vi "Unregister API.vi"(8 "error in (no error)":errorcluster, 10 "API":refnum<class "API.lvclass">, 11 "VolatusCore in":refnum<class "VolatusCoreTask.lvclass">) -> (0 "error out":errorcluster, 3 "VolatusCore out":refnum<class "VolatusCoreTask.lvclass">)   [LabVIEW 2020, in "Volatus.lvlib" / "VolatusCoreTask.lvclass"]
uses:
  VolatusCoreTask.lvclass
  API/API.lvclass
  VolatusCoreTask.lvclass/VolatusCoreTask.ctl
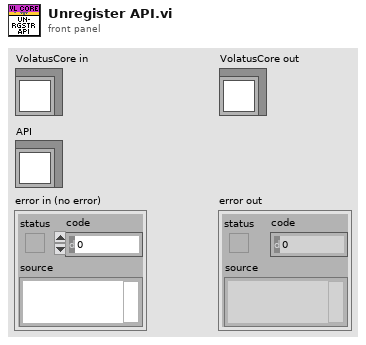
[diagram p1: front panel]
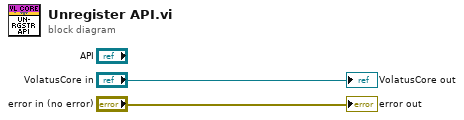
[diagram p0: block diagram]
diagram:
  "error out" <- "error in (no error)"
  "VolatusCore out" <- "VolatusCore in"
